vi "Initialize.vi"(8 "error in (no error)":errorcluster caption="Fehler (Eingang, kein Fehler)", 10 "Baud Rate":u32(ring) items=["9600 (default)", "19200", "38400", "57600", "115200"], 11 "input refnum":refnum<visa-resource-name> caption="Eingang (Referenz)") -> (0 "Cluster (Ausgang)":errorcluster, 3 "Referenz out":refnum<visa-resource-name>)   [LabVIEW 2013, in "PV ActiveLine.lvlib"]
doc: "The transmission rate of the USB interface is 115200 baud and can be changed.\n\nThe transmission rate of the RS485 interface is 9600 baud and cannot be changed."
uses:
  PV ActiveLine.lvlib
panel:
  in  "Buffer":u16=5000
  in  "Baud Rate 2":u32[](array[numeric])=[9600, 19200, 38400, 57600, 115200]
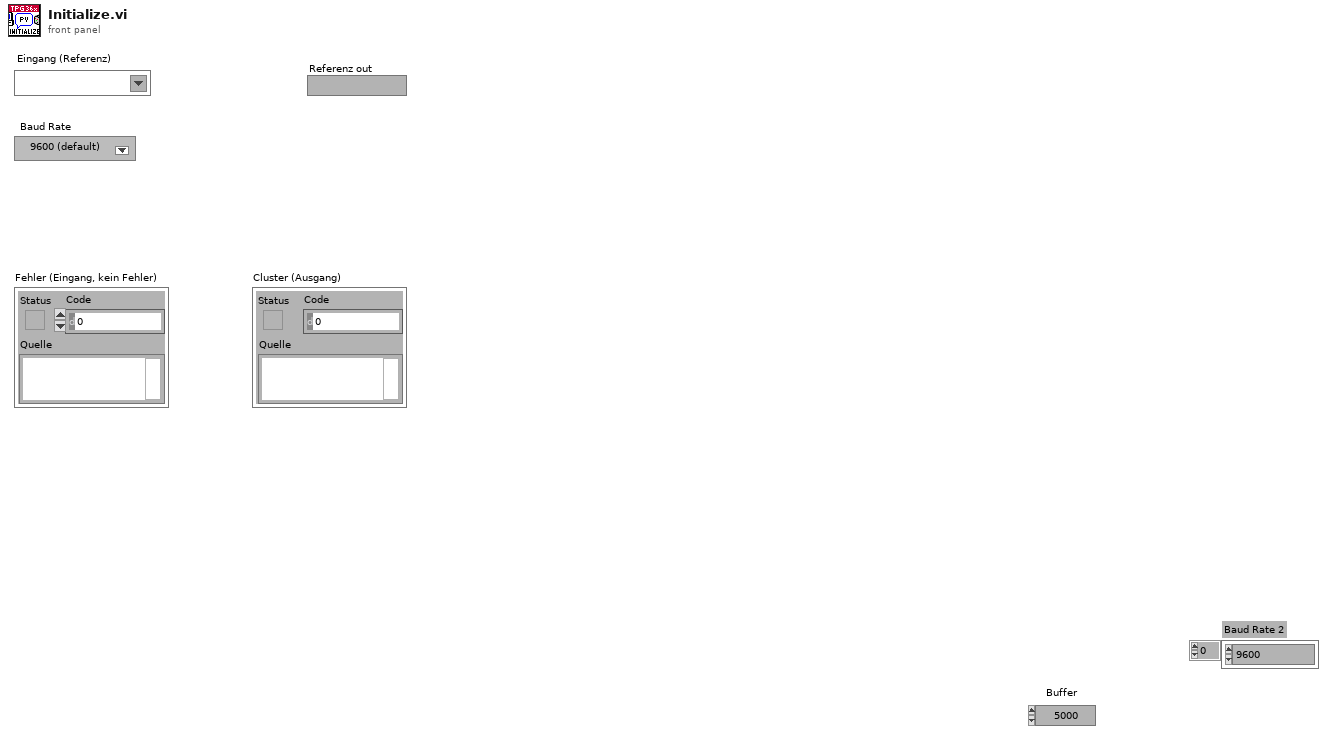
[diagram p1: front panel]
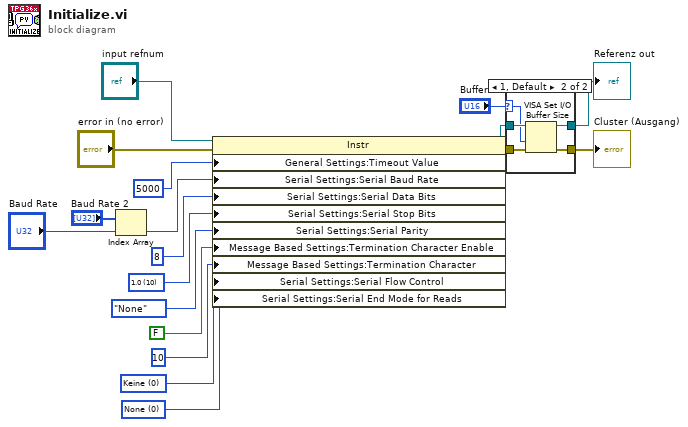
[diagram p0: block diagram]
diagram:
  w12 = u16 10 items=["1.0"=10, "1.5"=15, "2.0"=20] ("stop bits (10: 1 bit)")
  w14 = u16 0 items=["Keine", "XON/XOFF", "RTS/CTS", "XON/XOFF & RTS/CTS", "DTR/DSR", "XON/XOFF & DTR/DSR"] ("flow control (0:none)")
  w15 = u16 0 items=["None", "LastBit", "TermChar"] ("Serial Settings:Serial End Mode for Reads")
  n1 = Index Array(array="Baud Rate 2", index="Baud Rate") -> (element=w16:u32)
  n2 = property class="Instr"(reference="input refnum", error in="error in (no error)", "General Settings:Timeout Value"=u32 5000 ("timeout (10sec)"), "Serial Settings:Serial Baud Rate"=w16, "Serial Settings:Serial Data Bits"=u16 8 ("data bits (8)"), "Serial Settings:Serial Stop Bits"=w12, "Serial Settings:Serial Parity"=enum16{"None", "Odd", "Even", "Mark", "Space"}."None" ("parity (0:none)"), "Message Based Settings:Termination Character Enable"=FALSE ("Enable Termination\nChar (T)"), "Message Based Settings:Termination Character"=u8 10 ("termination char\n(0xA = '\\n' = LF)"), "Serial Settings:Serial Flow Control"=w14, "Serial Settings:Serial End Mode for Reads"=w15) -> (reference out=w17:refnum<visa-resource-name>, error out=w18:errorcluster)
  n3 = case shown="1, Default" "Buffer" {
    selector: "Buffer" -> [_ w24]
    tunnel: w17 -> [w19 w25]
    tunnel: w18 -> [w20 w21]
    tunnel: [w20 w23] -> w5
    tunnel: [w19 w22] -> w4
    frame 0 {
    }
    frame 1, Default {
      n4 = VISA Set I/O Buffer Size(VISA resource name=w25, size (4096)=w24, error in (no error)=w21) -> (VISA resource name out=w22:refnum<visa-resource-name>, error out=w23:errorcluster)  [unwired: 1 in]
    }
  }
  "Cluster (Ausgang)" <- w5
  "Referenz out" <- w4
